vi "Exception Throw.vi"(0 "message":string, 2 "Exception in":refnum<class "Exception.lvclass">, 11 "error in (no error)":errorcluster) -> (15 "error out":errorcluster)   [LabVIEW 2015, in "LV Exceptions v1.lvlib" / "Exception.lvclass"]
doc: "Initializes and inserts exception object into error cluster."
uses:
  Exception.lvclass
  Exception.lvclass/Exception.ctl
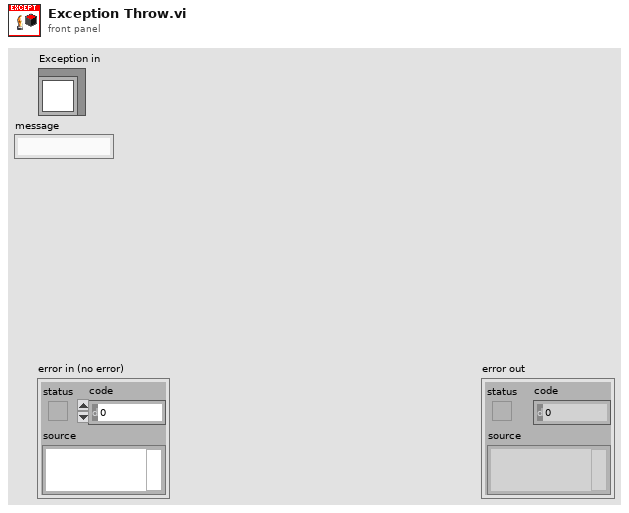
[diagram p1: front panel]
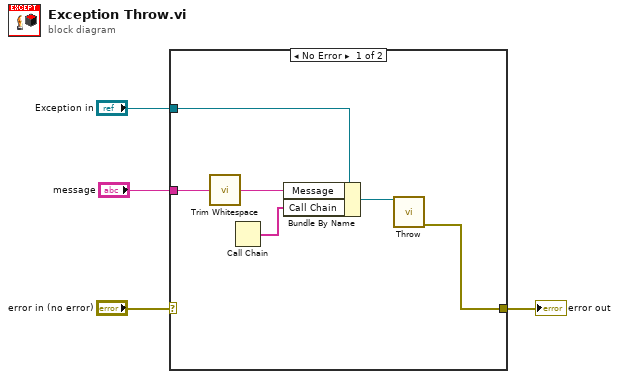
[diagram p0: block diagram]
diagram:
  n1 = case shown="No Error" "error in (no error)" {
    selector: "error in (no error)" -> [_ w11]
    tunnel: [w7 w11] -> w3
    tunnel: "Exception in" -> [w10 _]
    tunnel: "message" -> [w6 _]
    frame No Error {
      n2 = call <vilib>:"Trim Whitespace.vi"("string"=w6) -> ("trimmed string"=w5:string)  [unwired: 1 in]
      n3 = Call Chain() -> (call chain=w9:string[])
      n4 = Bundle By Name(cluster=w10, "Message"=w5, "Call Chain"=w9) -> (w8:refnum<class "Exception.lvclass">)
      n5 = call-dynamic "Throw.vi"("exception"=w8) -> ("error out"=w7:errorcluster)  [unwired: 13 in, 1 out]
    }
    frame Error {
    }
  }
  "error out" <- w3
